vi "Read ATML File.vi"() -> ()   [LabVIEW 2023]
doc: "Read the contents of an ATML file and display them."
uses:
  <vilib>/Platform/storage/lvStorage.llb/_openFunction.ctl
  <vilib>/Platform/storage/lvStorage.llb/_openStorageWithRootAutoDetect.vi
  <vilib>/Platform/storage/lvStorage.llb/xStorage/xStorageSupp/ErrorOut.vi
  <vilib>/Platform/storage/lvStorage.llb/_queryPropPoly.vi
  <vilib>/Platform/storage/lvStorage.llb/_queryPropString.vi
  <vilib>/Platform/storage/lvStorage.llb/_queryGenericObjects.vi
  <vilib>/Platform/storage/Storage.llb/Get Property (String).vi
  <vilib>/Platform/storage/Storage.llb/Get Object Info.vi
  <vilib>/Platform/storage/Storage.llb/__closeStorageFromObject.vi
  <vilib>/Platform/storage/lvStorage.llb/xStorage/Open Data Storage/Open Data Storage.xnode
  <vilib>/Platform/storage/lvStorage.llb/xStorage/Read Data/Read Data.xnode
  <vilib>/Platform/storage/lvStorage.llb/xStorage/Close Data Storage/Close Data Storage.xnode
panel:
  out "Numeric Limit Test Properties":string[][](table)
  # "Overview: Demonstrates the use of the DataPlugins VIs to read the contents of an ATML file, and convert it to a TDMS file.\nRequirements: Windows\nInstructions:\n1. Open Register ATML DataPlugin.vi and follow the instructions on its front panel.\n2. Run this VI. You should see  Data File Viewer to present the data.\n3. Quit the Data File Viewer. You should see string property data from the ATML file in the table below."
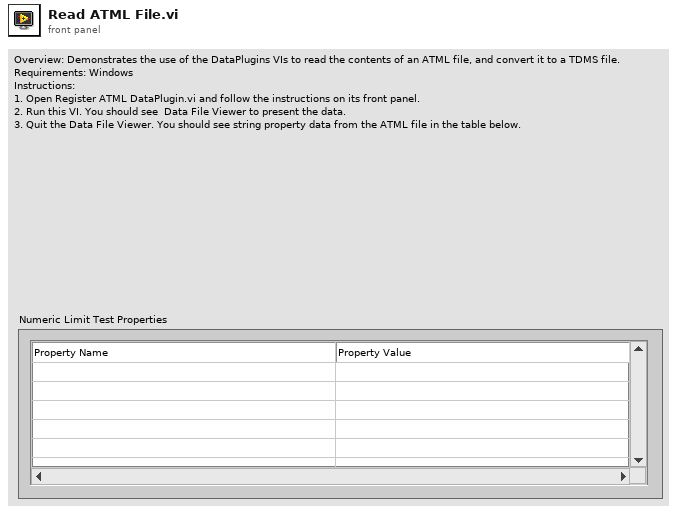
[diagram p1: front panel]
types:
  T1 = typedef "usiProperty.ctl" = cluster{"object type":T2, "property name":string, "data type":T3}
  T2 = typedef "usiObjectType.ctl" = enum16{"File", "Channel Group", "Channel", "Unknown"}
  T3 = typedef "usiDataType.ctl" = enum16{"eNoTypeUsi", "eInt8Usi", "eInt16Usi", "eInt32Usi", "eInt64Usi", "eUInt8Usi", "eUInt16Usi", "eUInt32Usi", "eUInt64Usi", "eFloat32Usi", "eFloat64Usi", "- 0", "- 1", "- 2", "- 3", "- 4", "- 5", "- 6", "- 7", "- 8", "- 9", "eString8Usi", "eString16Usi", "eStringUsi", "eEnumUsi", "- 10", "- 11", "- 12", "- 13", "- 14", "eTimeUsi", "- 15", "- 16", "- 17", "- 18", "- 19", "- 20", "- 21", "- 22", "- 23", "eInstanceUsi", "eStoreUsi"}
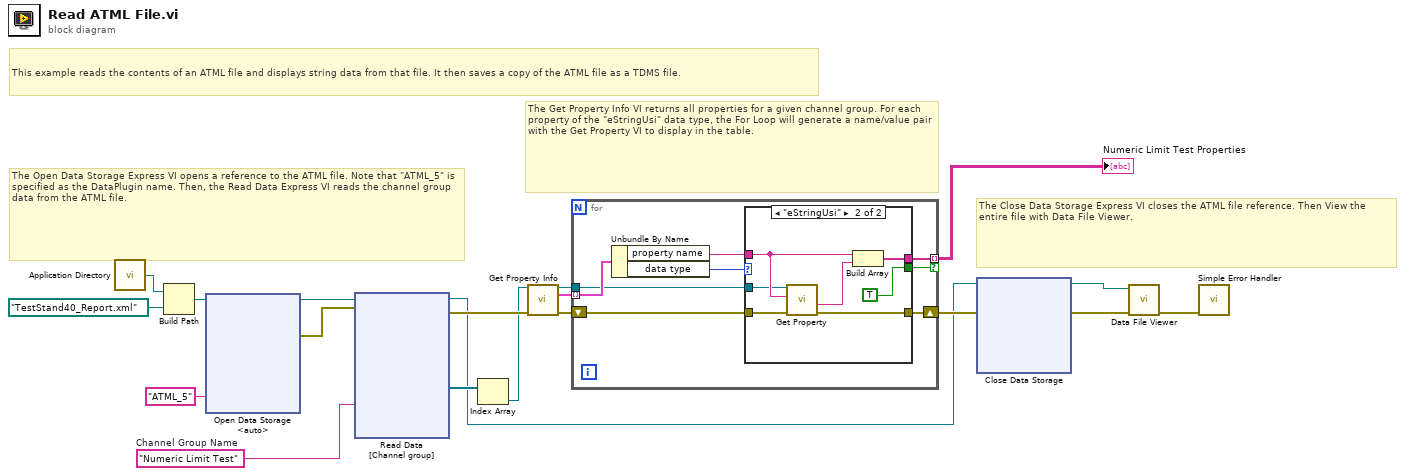
[diagram p0: block diagram]
diagram:
  w11 = "Numeric Limit Test"  # Channel Group Name
  # "The Close Data Storage Express VI closes the ATML file reference. Then View the entire file with Data File Viewer."
  # "The Get Property Info VI returns all properties for a given channel group. For each property of the \"eStringUsi\" data type, the For Loop will generate a name/value pair with the Get Property VI to display in the table."
  # "The Open Data Storage Express VI opens a reference to the ATML file. Note that \"ATML_5\" is specified as the DataPlugin name. Then, the Read Data Express VI reads the channel group data from the ATML file."
  # "This example reads the contents of an ATML file and displays string data from that file. It then saves a copy of the ATML file as a TDMS file."
  n1 = call <vilib>:"Application Directory.vi"() -> ("Application Directory"=w9:path)
  n2 = Build Path(base path=w9, name or relative path=path "TestStand40_Report.xml" ("file name")) -> (appended path=w19:path)
  n3 = xnode "Open Data Storage\n<auto>"("DataPlugin name"="ATML_5", "file path"=w19) -> ("storage refnum (file)"=w18:refnum<k20>, "error out"=w17:errorcluster)  [unwired: 3 in, 1 out]
  n4 = xnode "Read Data\n[Channel group]"("Name"=w11, "storage refnum (file)"=w18, "error in"=w17) -> ("storage refnums (channel group)"=w16:refnum<k20>[], "storage refnum (file) out"=w13:refnum<k20>, "error out"=w15:errorcluster)  [unwired: 1 in]
  n5 = Index Array(array=w16) -> (element=w4:refnum<k20>)  [unwired: 1 in]
  n6 = call <vilib>:"Get Property Info.vi"("storage refnum"=w4, "error in (no error)"=w15) -> ("storage refnum out"=w5:refnum<k20>, "properties"=w6:T1[], "error out"=w7:errorcluster)  [unwired: 11 in]
  n7 = for {
    shift-right: [w25] -> w14
    shift-left: w7 -> [w26]
    tunnel: w6 -> [w27] mode=indexing
    tunnel: w5 -> [w23]
    tunnel: [w22] -> w8 mode=indexing if=w21
    n8 = Unbundle By Name(w27) -> ("property name"=w24:string, "data type"=w20:T3)
    n9 = case shown="\"eStringUsi\"" w20 {
      tunnel: w26 -> [w28 w35]
      tunnel: [w28 w34] -> w25
      tunnel: w24 -> [_ w33]
      tunnel: w23 -> [_ w31]
      tunnel: [_ w30] -> w22
      tunnel: [_ TRUE] -> w21
      frame Default {
      }
      frame "eStringUsi" {
        n10 = call-poly <vilib>:"Get Property.vi"("error in (no error)"=w35, "Property name"=w33, "storage refnum"=w31) -> ("error out"=w34:errorcluster, "Value"=w32:string)  [unwired: 6 in, 1 out]
        n11 = Build Array(w33, w32) -> (w30:string[])
      }
    }
  }
  "Numeric Limit Test Properties" <- w8
  n12 = xnode "Close Data Storage\n"("storage refnum (file)"=w13, "error in (no error)"=w14) -> ("file path"=w3:path, "error out"=w2:errorcluster)
  n13 = call <vilib>:"Data File Viewer.vi"("error in (no error)"=w2, "file path"=w3) -> ("error out"=w1:errorcluster)  [unwired: 3 in, 2 out]
  n14 = call <vilib>:"Simple Error Handler.vi"("error in (no error)"=w1) -> ()  [unwired: 4 in, 5 out]
